vi "WPI_IMU_Loop.vi"(8 "error in":errorcluster, 11 "ADI IMU Interrupt DevRef":T1={"SimpleGyroDevRef"={"DevStatus"={"status"=FALSE, "code"=0, "source"=""}, "Handle"=0, "SPI Bus"=enum."SPI On-Board, CS0", "Device Found"=FALSE, "Sample Rate"=0.0, "Device Ready"=FALSE, "Yaw Axis"=enum."Z"}, "InterruptRef"={"DevStatus"={"status"=FALSE, "code"=0, "source"=""}, "InterruptIndex"=enum."0"}} {"SimpleGyroDevRef"."Sample Rate" min=0.25 max=100.0 step=0.25}) -> (0 "error out":errorcluster)   [LabVIEW 2015, in "FRC ADI MXP IMU.lvlib"]
doc: "Periodically reads the ADI MXP IMU valuse and makes data available for use elsewhere in your robot project. Place this block within PeriodicTasks.vi outside any loops."
uses:
  FRC ADI MXP IMU.lvlib
  WPI_AnalogDevicesIMUInterruptDevRef.ctl
  WPI_AnalogDevicesIMUDevRef.ctl
  <vilib>/Rock Robotics/SystemInterfaces/spilib/spi_bus.ctl
  <vilib>/Rock Robotics/WPI/Interrupt/WPI_InterruptRef.ctl
  <vilib>/Rock Robotics/SystemInterfaces/Interrupt/FPGA_InterruptIndex.ctl
  <vilib>/Rock Robotics/WPI/SPI/WPI_SPIDevRef.ctl
  <vilib>/Platform/TimedLoop/XDataNode/timing_clust.ctl
  <vilib>/Platform/TimedLoop/XDataNode/nitl_modes.ctl
  <vilib>/Platform/TimedLoop/XDataNode/wakeup.ctl
  <vilib>/Rock Robotics/SystemInterfaces/Interrupt/FPGA_WaitOnInterrupt.vi
  <vilib>/Rock Robotics/WPI/Utilities/WPI_UtilitiesTimebaseConstants.vi
  <vilib>/Rock Robotics/SystemInterfaces/Interrupt/FPGA_InterruptReadTimestamp.vi
  <vilib>/platform/TimedLoop/XDataNode/XDataNode.xnode
  <vilib>/ptbypt/NI_PtbyPt.lvlib
  <vilib>/Platform/TimedLoop/XDataNode/XDNodeRunTimeDep.lvlib
panel:
  out "Device Found":bool
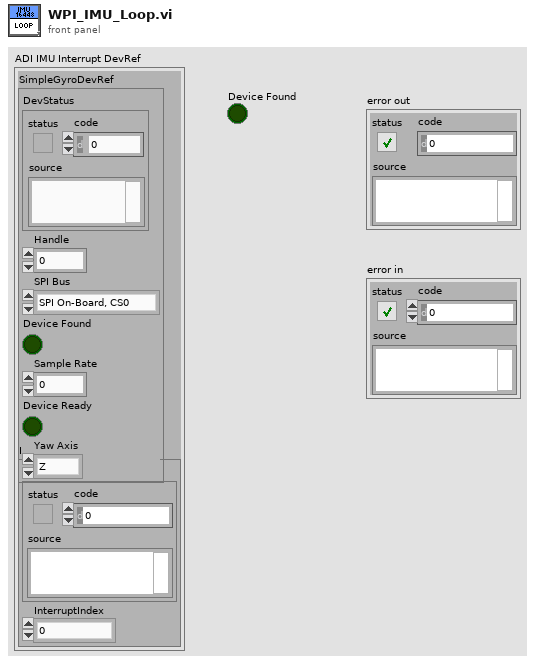
[diagram p1: front panel]
types:
  T1 = typedef "FRC ADI MXP IMU.lvlib/WPI_AnalogDevicesIMUInterruptDevRef.ctl" = cluster{"SimpleGyroDevRef":T2, "InterruptRef":T4}
  T2 = typedef "FRC ADI MXP IMU.lvlib/WPI_AnalogDevicesIMUDevRef.ctl" = cluster{"DevStatus":errorcluster, "Handle":i32, "SPI Bus":T3, "Device Found":bool, "Sample Rate":dbl, "Device Ready":bool, "Yaw Axis":enum16{"X", "Y", "Z"}}
  T3 = typedef "spi_bus.ctl" = enum16{"SPI On-Board, CS0", "SPI On-Board, CS1", "SPI On-Board, CS2", "SPI On-Board, CS3", "SPI MXP", "Invalid"}
  T4 = typedef "WPI_InterruptRef.ctl" = cluster{"DevStatus":errorcluster, "InterruptIndex":T5}
  T5 = typedef "FPGA_InterruptIndex.ctl" = enum8{"0", "1", "2", "3", "4", "5", "6", "7", "Invalid"}
  T6 = typedef "WPI_SPIDevRef.ctl" = cluster{"DevStatus":errorcluster, "Handle":i32, "SPI Bus":T3}
  T7 = cluster{"Output[0]":dbl, "Output[1]":dbl, "Output[2]":dbl}
  T8 = typedef "XDNodeRunTimeDep.lvlib/timing_clust.ctl" = cluster{"Expected End [f-1]":u64, "Actual End [f-1]":u64, "Finished Late? [f-1]":bool, "Expected End [i-1]":u64, "Actual End [i-1]":u64, "Finished Late? [i-1]":bool, "Expected Start [i]":u64, "Actual Start [i]":u64, "Expected Start [f]":u64, "Actual Start [f]":u64, "Source Name":string, "Structure Name":string, "Period":i64, "Deadline":i64, "Offset":i64, "Start":i64, "Priority":i32, "Timeout":i32, "Mode":T9, "Wakeup Reason":T10, "Error":errorcluster, "Source Type":string, "Secondary Source Type":string, "Global End Time":u64, "Global Start Time":u64, "Frame Duration":u64, "Iteration Duration":u64, "Assigned CPU":i32, "I/O Scan Engine Mode":u32}
  T9 = typedef "XDNodeRunTimeDep.lvlib/nitl_modes.ctl" = enum32{"No Change", "Process missed periods, maintain original phase", "Discard missed periods, maintain original phase", "Process missed periods, ignore original phase", "Discard missed periods, ignore original phase"}
  T10 = typedef "XDNodeRunTimeDep.lvlib/wakeup.ctl" = enum32{"Normal", "Aborted", "Asynchronous wakeup", "Timing source error", "Timed loop error", "Timeout"}
  T11 = cluster{"Data Array[0]":dbl, "Data Array[1]":dbl, "Data Array[2]":dbl, "Data Array[3]":dbl, "Data Array[4]":dbl, "Data Array[5]":dbl, "Data Array[6]":dbl, "Data Array[7]":dbl, "Data Array[8]":dbl, "Data Array[9]":dbl, "Data Array[10]":dbl}
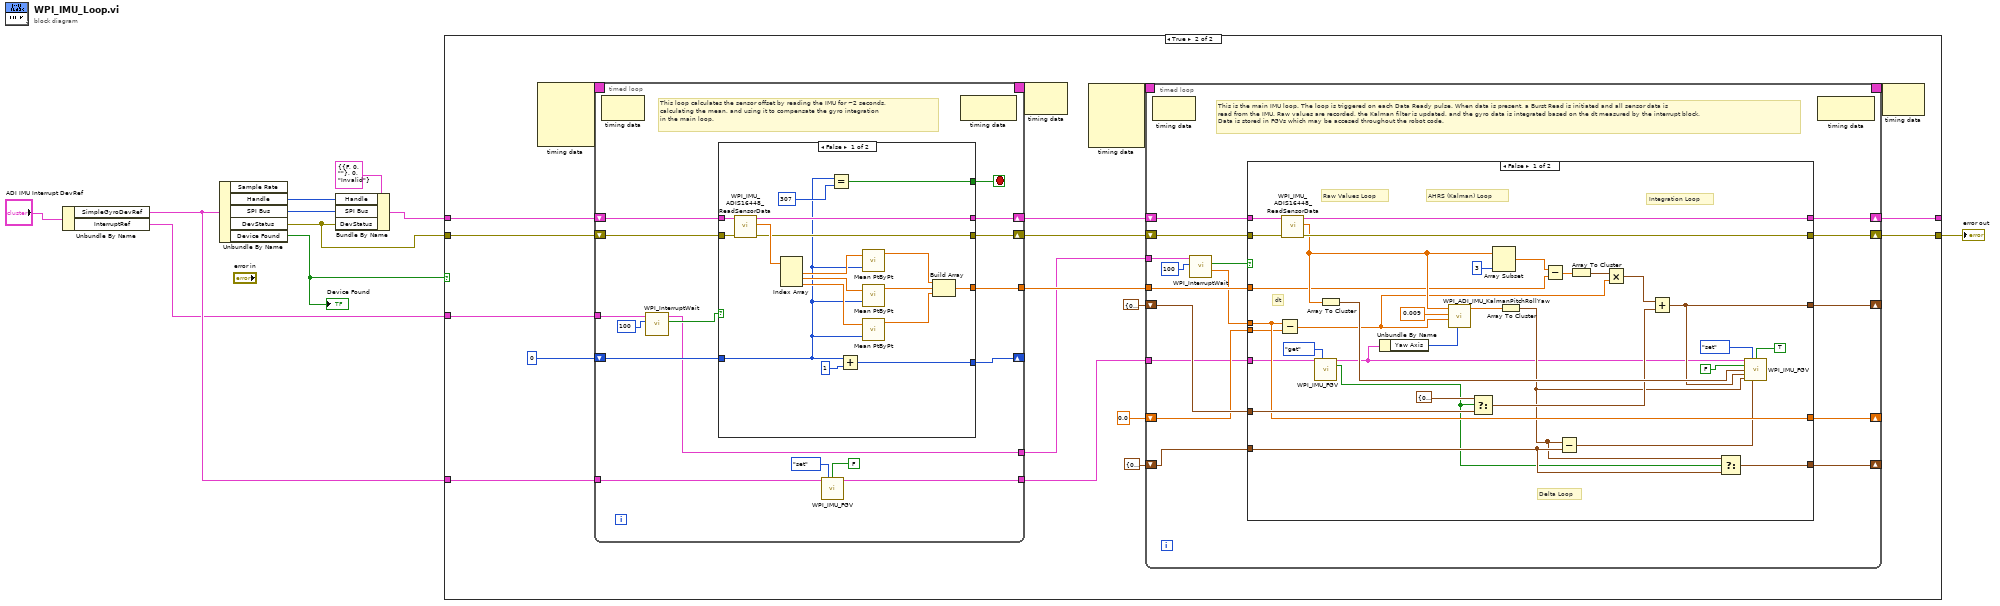
[diagram p0: block diagram]
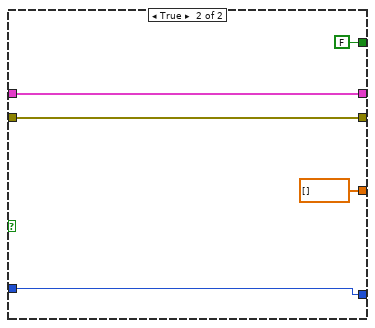
[diagram p4: hidden frame]
diagram:
  n1 = Unbundle By Name("ADI IMU Interrupt DevRef") -> ("SimpleGyroDevRef"=w2:T2, "InterruptRef"=w1:T4)
  n2 = Unbundle By Name(w2) -> ("Handle"=w9:i32, "SPI Bus"=w8:T3, "DevStatus"=w5:errorcluster, "Device Found"=w7:bool)  [unwired: 1 out]
  "Device Found" <- w7
  n3 = Bundle By Name(cluster=T6 {"DevStatus"={"status"=FALSE, "code"=0, "source"=""}, "Handle"=0, "SPI Bus"=enum."Invalid"} ("SPIDevRef out"), "Handle"=w9, "SPI Bus"=w8, "DevStatus"=w5) -> (w6:T6)
  n4 = case shown="True" w7 {
    tunnel: w6 -> [w12 w29]
    tunnel: w5 -> [w11 w28]
    tunnel: [w11 w31] -> w4
    tunnel: [w12 w30] -> _
    tunnel: w2 -> [_ w16]
    tunnel: w1 -> [_ w18]
    frame False {
    }
    frame True {
      n5 = node-c288() -> (w20:T8)  [unwired: 4 in]
      n6 = timed-loop {
        tunnel: [w103] -> w24
        shift-right: [w105] -> w26
        shift-left: w29 -> [w97]
        shift-right: [w106] -> w27
        shift-left: w28 -> [w96]
        shift-right: [w101] -> _
        shift-left: 0 -> [w102]
        tunnel: w18 -> [w100]
        tunnel: [w95] -> w22
        timing: w20 -> [_]
        timing-out: [_] -> w19
        tunnel: w16 -> [w93]
        tunnel: [w94] -> w13
        stop <- w104 stop-if-true
        # "This loop calculates the sensor offset by reading the IMU for ~2 seconds, \ncalculating the mean, and using it to compensate the gyro integration\nin the main loop."
        n7 = node-c288() -> ()  [unwired: 1 in, 1 out]
        n8 = call <vilib>:"WPI_InterruptWait.vi"("Timeout (ms)"=100, "InterruptRef"=w100) -> ("Timed Out"=w98:bool, "InterruptRef"=w95:T4)  [unwired: 5 in, 3 out]
        n9 = case shown="False" w98 {
          tunnel: [w124 w127] -> w106
          tunnel: [w123 w128] -> w105
          tunnel: [w118 FALSE] -> w104
          tunnel: [w114 dbl[] []] -> w103
          tunnel: w96 -> [w113 w127]
          tunnel: w97 -> [w112 w128]
          tunnel: w102 -> [w109 w130]
          tunnel: [w111 w130] -> w101
          frame False {
            n10 = call "WPI_IMU_ADIS16448_ReadSensorData.vi"("error in (no error)"=w113, "SPIDevRef in"=w112) -> ("error out"=w124:errorcluster, "Data Array"=w125:dbl[], "SPIDevRef out"=w123:T6)  [unwired: 7 in]
            n11 = Index Array(array=w125) -> (element #1=w122:dbl, element #2=w121:dbl, element #3=w120:dbl)  [unwired: 3 in]
            n12 = Equal?(x=w109, y=307) -> (x = y?=w118:bool)
            n13 = Add(x=w109, y=1) -> (x+y=w111:i32)
            n14 = call <vilib>:"Mean PtByPt.vi"("x"=w122, "sample length"=w109) -> ("mean"=w117:dbl)  [unwired: 2 in, 1 out]
            n15 = call <vilib>:"Mean PtByPt.vi"("x"=w121, "sample length"=w109) -> ("mean"=w116:dbl)  [unwired: 2 in, 1 out]
            n16 = call <vilib>:"Mean PtByPt.vi"("x"=w120, "sample length"=w109) -> ("mean"=w115:dbl)  [unwired: 2 in, 1 out]
            n17 = Build Array(w117, w116, w115) -> (w114:dbl[])
          }
          frame True {
          }
        }
        n18 = call "WPI_IMU_FGV.vi"("SimpleGyroDevRef"=w93, "Operation"=enum16{"set", "get"}."set", "Sensor Ready?"=FALSE) -> ("SimpleGyroDevRef"=w94:T2)  [unwired: 6 in, 6 out]
        n19 = node-c288() -> ()  [unwired: 1 in, 1 out]
      }
      n20 = node-c288(w19) -> ()  [unwired: 1 out]
      n21 = node-c288() -> (w15:T8)  [unwired: 4 in]
      n22 = timed-loop {
        shift-right: [w48] -> w30
        shift-left: w26 -> [w42]
        shift-right: [w47] -> w31
        shift-left: w27 -> [w41]
        shift-right: [w45] -> _
        shift-left: cluster{dbl, dbl, dbl} {0.0, 0.0, 0.0} -> [w44]
        tunnel: w24 -> [w43]
        tunnel: w22 -> [w39]
        shift-right: [w37] -> _
        shift-left: 0.0 ("TimeStamp") -> [w36]
        shift-right: [w33] -> _
        shift-left: T7 {"Output[0]"=0.0, "Output[1]"=0.0, "Output[2]"=0.0} -> [w35]
        tunnel: w13 -> [w32]
        timing: w15 -> [_]
        timing-out: [_] -> w14
        stop <- FALSE stop-if-true
        # "This is the main IMU loop. The loop is triggered on each Data Ready pulse. When data is present, a Burst Read is initiated and all sensor data is \nread from the IMU. Raw values are recorded, the Kalman filter is updated, and the gyro data is integrated based on the dt measured by the interrupt block.\nData is stored in FGVs which may be accesed throughout the robot code."
        n23 = node-c288() -> ()  [unwired: 1 in, 1 out]
        n24 = call <vilib>:"WPI_InterruptWait.vi"("Timeout (ms)"=100, "InterruptRef"=w39) -> ("TimeStamp"=w38:dbl, "Timed Out"=w34:bool)  [unwired: 5 in, 3 out]
        n25 = case shown="False" w34 {
          tunnel: w42 -> [w83 w88]
          tunnel: w41 -> [w82 w87]
          tunnel: [w81 w88] -> w48
          tunnel: [w80 w87] -> w47
          tunnel: w32 -> [w55 _]
          tunnel: [w69 w86] -> w45
          tunnel: w44 -> [w73 w86]
          tunnel: w43 -> [w67 _]
          tunnel: w38 -> [w63 _]
          tunnel: [w63 w85] -> w37
          tunnel: w36 -> [w62 w85]
          tunnel: w35 -> [w59 w84]
          tunnel: [w58 w84] -> w33
          frame False {
            # "Delta Loop"
            # "dt"
            # "Integration Loop"
            # "AHRS (Kalman) Loop"
            # "Raw Values Loop"
            n26 = Subtract(x=w63, y=w62) -> (x-y=w61:dbl)
            n27 = call "WPI_IMU_ADIS16448_ReadSensorData.vi"("error in (no error)"=w82, "SPIDevRef in"=w83) -> ("error out"=w80:errorcluster, "Data Array"=w71:dbl[], "SPIDevRef out"=w81:T6)  [unwired: 7 in]
            n28 = call "WPI_IMU_FGV.vi"("SimpleGyroDevRef"=w55, "Operation"=enum16{"set", "get"}."get") -> ("SimpleGyroDevRef"=w52:T2, "Reset Out"=w54:bool)  [unwired: 7 in, 5 out]
            n29 = Array To Cluster(array=w71) -> (cluster=w77:T11)
            n30 = Unbundle By Name(w52) -> ("Yaw Axis"=w51:enum16{"X", "Y", "Z"})
            n31 = call "WPI_ADI_IMU_KalmanPitchRollYaw.vi"("Yaw Axis"=w51, "dt (s)"=w61, "Beta"=0.009, "Data"=w71) -> ("Output"=w76:dbl[])  [unwired: 7 in]
            n32 = Select(t=T7 {"Output[0]"=0.0, "Output[1]"=0.0, "Output[2]"=0.0} ("cluster"), s=w54, f=w73) -> (s? t:f=w72:T7)
            n33 = Array Subset(array=w71, length=3) -> (w68:dbl[])  [unwired: 1 in]
            n34 = Array To Cluster(array=w76) -> (cluster=w57:T7)
            n35 = Subtract(x=w68, y=w67) -> (x-y=w66:dbl[])
            n36 = Subtract(x=w57, y=w59) -> (x-y=w60:T7)
            n37 = Array To Cluster(array=w66) -> (cluster=w65:cluster{"[0]":dbl, "[1]":dbl, "[2]":dbl})
            n38 = Multiply(x=w65, y=w61) -> (x*y=w64:cluster{"[0]":dbl, "[1]":dbl, "[2]":dbl})
            n39 = Add(x=w64, y=w72) -> (x+y=w69:cluster{dbl, dbl, dbl})
            n40 = Select(t=w57, s=w54, f=w59) -> (s? t:f=w58:T7)
            n41 = call "WPI_IMU_FGV.vi"("SimpleGyroDevRef"=w52, "Operation"=enum16{"set", "get"}."set", "Sensor Ready?"=TRUE, "Reset"=FALSE ("Calibrated"), "IMU Data"=w77, "IMU Angles"=w69, "IMU AHRS"=w57, "IMU AHRS DELTA"=w60) -> ()  [unwired: 1 in, 7 out]
          }
          frame True {
            # "Waiting for an interrupt..."
          }
        }
        n42 = node-c288() -> ()  [unwired: 1 in, 1 out]
      }
      n43 = node-c288(w14) -> ()  [unwired: 1 out]
    }
  }
  "error out" <- w4
